vi "Operational Force Test SAA.vi"(8 "error in (no error)":errorcluster, 10 "Model in":refnum<class "Model.lvclass">, 11 "Test Actuator State in":refnum<class "Test Actuator State.lvclass">) -> (0 "error out":errorcluster, 1 "Pass":bool, 2 "Model out":refnum<class "Model.lvclass">, 3 "Test Actuator State out":refnum<class "Test Actuator State.lvclass">)   [LabVIEW 2016]
uses:
  Model/Model/Model.lvclass
  Typedefs/ActuatorSetPoints.ctl
  <vilib>/platform/TimedLoop/XDataNode/XDataNode.xnode
  <vilib>/Platform/TimedLoop/XDataNode/nitl_modes.ctl
  <vilib>/Platform/TimedLoop/XDataNode/XDNodeRunTimeDep.lvlib
  <vilib>/Platform/TimedLoop/XDataNode/wakeup.ctl
  <vilib>/Platform/TimedLoop/XDataNode/timing_clust.ctl
  Test Actuator State.lvclass
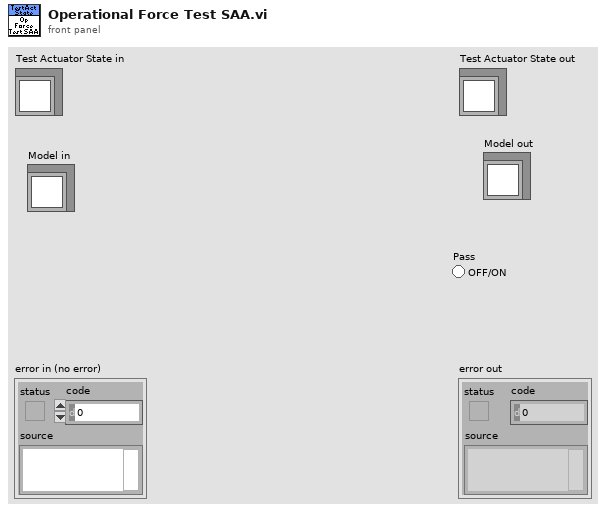
[diagram p1: front panel]
types:
  T1 = typedef "ForcePair.ctl" = cluster{"Axial Force":dbl, "Lateral Force":dbl}
  T2 = typedef "OperationalForceTestSettings.ctl" = cluster{"Max Force Error (N)":dbl, "Max Moment (NM)":dbl, "Process Time (s)":dbl, "Sample Time (s)":dbl}
  T3 = typedef "ActuatorSetPoints.ctl" = cluster{"Axial Force":dbl, "Lateral Force":dbl, "FC1 Force":dbl, "FC2 Force":dbl}
  T4 = typedef "XDNodeRunTimeDep.lvlib/timing_clust.ctl" = cluster{"Expected End [f-1]":u64, "Actual End [f-1]":u64, "Finished Late? [f-1]":bool, "Expected End [i-1]":u64, "Actual End [i-1]":u64, "Finished Late? [i-1]":bool, "Expected Start [i]":u64, "Actual Start [i]":u64, "Expected Start [f]":u64, "Actual Start [f]":u64, "Source Name":string, "Structure Name":string, "Period":i64, "Deadline":i64, "Offset":i64, "Start":i64, "Priority":i32, "Timeout":i32, "Mode":T5, "Wakeup Reason":T6, "Error":errorcluster, "Source Type":string, "Secondary Source Type":string, "Global End Time":u64, "Global Start Time":u64, "Frame Duration":u64, "Iteration Duration":u64, "Assigned CPU":i32, "I/O Scan Engine Mode":u32}
  T5 = typedef "XDNodeRunTimeDep.lvlib/nitl_modes.ctl" = enum32{"No Change", "Process missed periods, maintain original phase", "Discard missed periods, maintain original phase", "Process missed periods, ignore original phase", "Discard missed periods, ignore original phase"}
  T6 = typedef "XDNodeRunTimeDep.lvlib/wakeup.ctl" = enum32{"Normal", "Aborted", "Asynchronous wakeup", "Timing source error", "Timed loop error", "Timeout"}
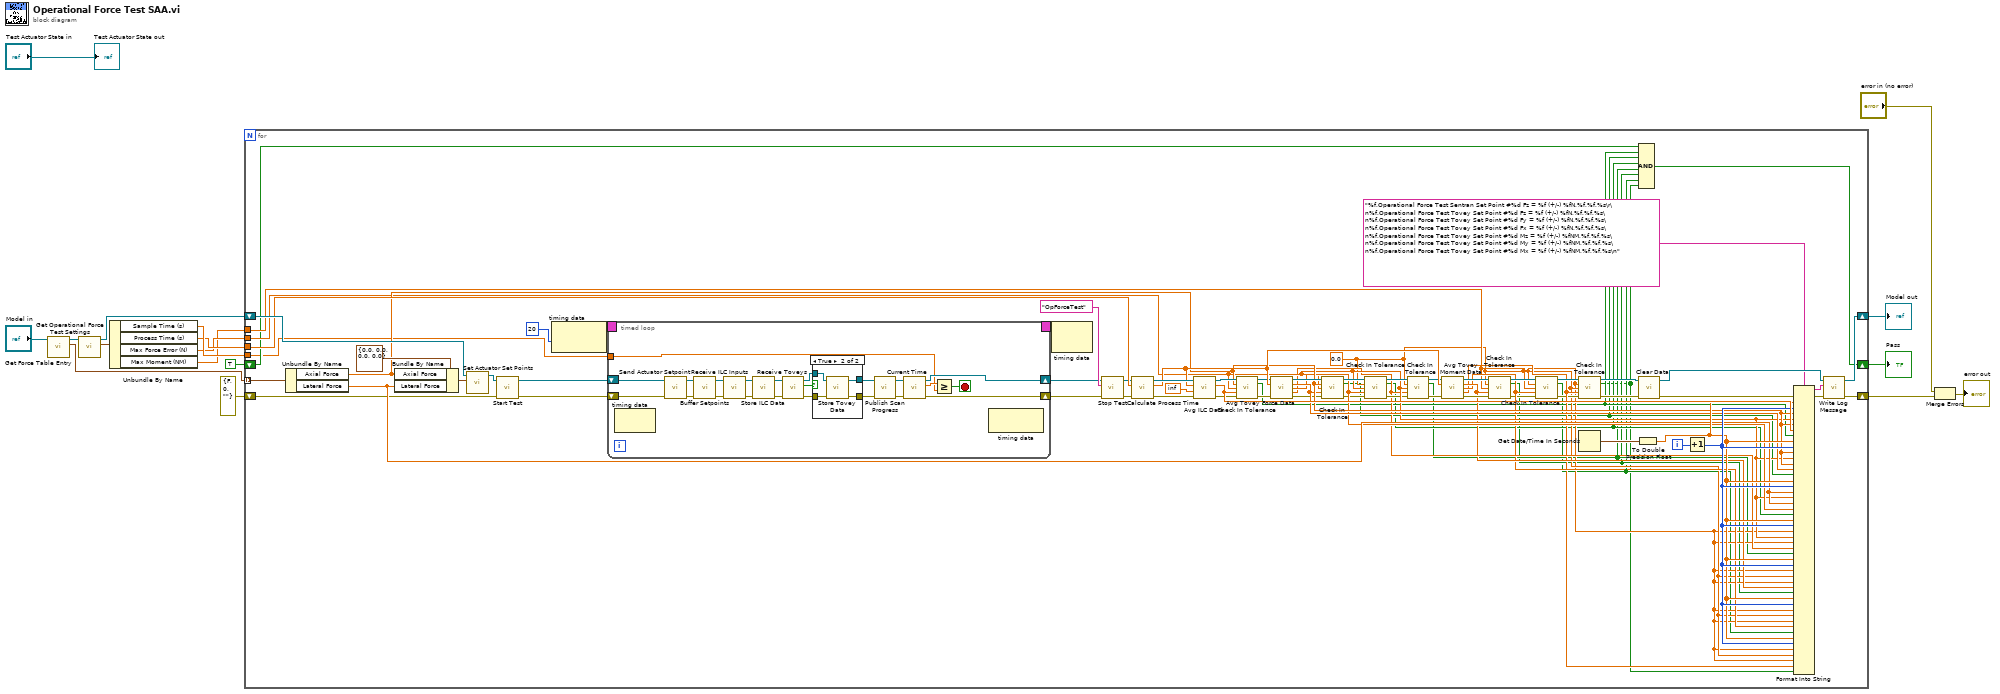
[diagram p0: block diagram]
diagram:
  n1 = call "Get Force Table Entry.vi"("Model in"="Model in") -> ("Entry"=w4:T1[], "Model out"=w7:refnum<class "Model.lvclass">)  [unwired: 8 in, 1 out]
  n2 = call-dynamic "Get Operational Force Test Settings.vi"("Model in"=w7) -> ("Operational Force Test Settings"=w5:T2, "Model out"=w6:refnum<class "Model.lvclass">)  [unwired: 9 in]
  n3 = Unbundle By Name(w5) -> ("Sample Time (s)"=w16:dbl, "Process Time (s)"=w15:dbl, "Max Force Error (N)"=w14:dbl, "Max Moment (NM)"=w9:dbl)
  n4 = for {
    tunnel: w4 -> [w83] mode=indexing
    shift-right: [w88] -> w11
    shift-left: w6 -> [w90]
    tunnel: w16 -> [w22]
    tunnel: w15 -> [w78]
    tunnel: w14 -> [w62]
    shift-right: [w79] -> w10
    shift-left: errorcluster {"status"=FALSE, "code"=0, "source"=""} ("error out") -> [w39]
    tunnel: w9 -> [w44]
    shift-right: [w29] -> w1
    shift-left: TRUE -> [w37]
    i -> [w85]
    w43 = 0.0
    n5 = Unbundle By Name(w83) -> ("Axial Force"=w68:dbl, "Lateral Force"=w65:dbl)
    n6 = Bundle By Name(cluster=T3 {"Axial Force"=0.0, "Lateral Force"=0.0, "FC1 Force"=0.0, "FC2 Force"=0.0} ("Actuator Set Points"), "Axial Force"=w68, "Lateral Force"=w65) -> (w84:T3)
    n7 = call "Set Actuator Set Points.vi"("Actuator Set Points"=w84, "Model in"=w90) -> ("Model out"=w38:refnum<class "Model.lvclass">)  [unwired: 9 in]
    n8 = call "Start Test.vi"("error in (no error)"=w39, "Model in"=w38) -> ("error out"=w20:errorcluster, "Model out"=w21:refnum<class "Model.lvclass">)  [unwired: 8 in]
    n9 = node-c288(i64 20 ("Period")) -> (w25:T4)
    n10 = timed-loop {
      timing: w25 -> [_]
      timing-out: [_] -> w24
      shift-right: [w95] -> w18
      shift-left: w20 -> [w96]
      shift-right: [w93] -> w19
      shift-left: w21 -> [w94]
      tunnel: w22 -> [w92]
      stop <- w97 stop-if-true
      n11 = node-c288() -> ()  [unwired: 1 in, 1 out]
      n12 = call "Send Actuator Setpoint.vi"("error in (no error)"=w96, "Model in"=w94) -> ("error out"=w112:errorcluster, "Model out"=w110:refnum<class "Model.lvclass">)  [unwired: 8 in]
      n13 = call "Buffer Setpoints.vi"("error in (no error)"=w112, "Model in"=w110) -> ("error out"=w113:errorcluster, "Model out"=w111:refnum<class "Model.lvclass">)  [unwired: 8 in]
      n14 = call "Receive ILC Inputs.vi"("error in (no error)"=w113, "Model in"=w111) -> ("error out"=w99:errorcluster, "Model out"=w98:refnum<class "Model.lvclass">)  [unwired: 8 in]
      n15 = call "Store ILC Data.vi"("error in (no error)"=w99, "Model in"=w98) -> ("error out"=w102:errorcluster, "Model out"=w101:refnum<class "Model.lvclass">)  [unwired: 8 in]
      n16 = call "Receive Toveys.vi"("error in (no error)"=w102, "Model in"=w101) -> ("error out"=w104:errorcluster, "Data Received"=w105:bool, "Model out"=w103:refnum<class "Model.lvclass">)  [unwired: 7 in]
      n17 = case shown="True" w105 {
        tunnel: w103 -> [w115 w119]
        tunnel: w104 -> [w114 w118]
        tunnel: [w114 w117] -> w109
        tunnel: [w115 w116] -> w106
        frame False {
        }
        frame True {
          n18 = call "Store Tovey Data.vi"("error in (no error)"=w118, "Model in"=w119) -> ("error out"=w117:errorcluster, "Model out"=w116:refnum<class "Model.lvclass">)  [unwired: 8 in]
        }
      }
      n19 = call "Publish Scan Progress.vi"("error in (no error)"=w109, "Model in"=w106) -> ("error out"=w108:errorcluster, "Model out"=w107:refnum<class "Model.lvclass">)  [unwired: 8 in]
      n20 = call "Current Time.vi"("error in (no error)"=w108, "Model in"=w107) -> ("error out"=w95:errorcluster, "Time"=w100:dbl, "Model out"=w93:refnum<class "Model.lvclass">)  [unwired: 7 in]
      n21 = Greater Or Equal?(x=w100, y=w92) -> (x >= y?=w97:bool)
      n22 = node-c288() -> ()  [unwired: 1 in, 1 out]
    }
    n23 = node-c288(w24) -> ()  [unwired: 1 out]
    n24 = call "Stop Test.vi"("error in (no error)"=w18, "Test"="OpForceTest", "Model in"=w19) -> ("error out"=w27:errorcluster, "Model out"=w28:refnum<class "Model.lvclass">)  [unwired: 7 in]
    n25 = call "Calculate Process Time.vi"("error in (no error)"=w27, "Seconds"=w78, "Model in"=w28) -> ("error out"=w76:errorcluster, "Time"=w75:dbl, "Model out"=w77:refnum<class "Model.lvclass">)  [unwired: 6 in]
    n26 = call "Avg ILC Data.vi"("error in (no error)"=w76, "Before This Time"=inf, "After This Time"=w75, "Model in"=w77) -> ("error out"=w72:errorcluster, "Force"=w73:dbl, "Model out"=w74:refnum<class "Model.lvclass">)  [unwired: 5 in]
    n27 = call "Check In Tolerance.vi"("Model in"=w74, "Expected"=w68, "Tolerance"=w62, "Actual"=w73, "error in (no error)"=w72) -> ("Model out"=w42:refnum<class "Model.lvclass">, "Pass"=w36:bool, "error out"=w41:errorcluster)  [unwired: 8 in]
    n28 = call "Avg Tovey Force Data.vi"("Model in"=w42, "After This Time"=w75, "error in (no error)"=w41) -> ("Model out"=w69:refnum<class "Model.lvclass">, "Fz"=w67:dbl, "Fy"=w64:dbl, "Fx"=w54:dbl, "error out"=w61:errorcluster)  [unwired: 8 in]
    n29 = call "Check In Tolerance.vi"("Model in"=w69, "Expected"=w68, "Tolerance"=w62, "Actual"=w67, "error in (no error)"=w61) -> ("Model out"=w66:refnum<class "Model.lvclass">, "Pass"=w35:bool, "error out"=w60:errorcluster)  [unwired: 8 in]
    n30 = call "Check In Tolerance.vi"("Model in"=w66, "Expected"=w43, "Tolerance"=w62, "Actual"=w64, "error in (no error)"=w60) -> ("Model out"=w63:refnum<class "Model.lvclass">, "Pass"=w34:bool, "error out"=w59:errorcluster)  [unwired: 8 in]
    n31 = call "Check In Tolerance.vi"("Model in"=w63, "Expected"=w43, "Tolerance"=w62, "Actual"=w54, "error in (no error)"=w59) -> ("Model out"=w57:refnum<class "Model.lvclass">, "Pass"=w33:bool, "error out"=w58:errorcluster)  [unwired: 8 in]
    n32 = call "Avg Tovey Moment Data.vi"("Model in"=w57, "After This Time"=w75, "error in (no error)"=w58) -> ("Model out"=w56:refnum<class "Model.lvclass">, "Mz"=w53:dbl, "My"=w50:dbl, "Mx"=w49:dbl, "error out"=w55:errorcluster)  [unwired: 8 in]
    n33 = call "Check In Tolerance.vi"("Model in"=w56, "Expected"=w43, "Tolerance"=w44, "Actual"=w53, "error in (no error)"=w55) -> ("Model out"=w52:refnum<class "Model.lvclass">, "Pass"=w32:bool, "error out"=w47:errorcluster)  [unwired: 8 in]
    n34 = call "Check In Tolerance.vi"("Model in"=w52, "Expected"=w43, "Tolerance"=w44, "Actual"=w50, "error in (no error)"=w47) -> ("Model out"=w51:refnum<class "Model.lvclass">, "Pass"=w31:bool, "error out"=w46:errorcluster)  [unwired: 8 in]
    n35 = call "Check In Tolerance.vi"("Model in"=w51, "Expected"=w43, "Tolerance"=w44, "Actual"=w49, "error in (no error)"=w46) -> ("Model out"=w48:refnum<class "Model.lvclass">, "Pass"=w30:bool, "error out"=w45:errorcluster)  [unwired: 8 in]
    n36 = Get Date/Time In Seconds() -> (seconds since 1Jan1904=w86:timestamp)
    n37 = To Double Precision Float(number=w86) -> (double precision float=w70:dbl)
    n38 = call "Clear Data.vi"("error in (no error)"=w45, "Model in"=w48) -> ("error out"=w81:errorcluster, "Model out"=w89:refnum<class "Model.lvclass">)  [unwired: 8 in]
    n39 = Compound Arithmetic op=AND(w37, w36, w35, w34, w33, w32, w31, w30) -> (w29:bool)
    n40 = Increment(x=w85) -> (x+1=w71:i32)
    n41 = Format Into String(format string="%f,Operational Force Test Sentran Set Point #%d Fz = %f (+/-) %fN,%f,%f,%s\r\n%f,Operational Force Test Tovey Set Point #%d Fz = %f (+/-) %fN,%f,%f,%s\n%f,Operational Force Test Tovey Set Point #%d Fy = %f (+/-) %fN,%f,%f,%s\n%f,Operational Force Test Tovey Set Point #%d Fx = %f (+/-) %fN,%f,%f,%s\n%f,Operational Force Test Tovey Set Point #%d Mz = %f (+/-) %fNM,%f,%f,%s\n%f,Operational Force Test Tovey Set Point #%d My = %f (+/-) %fNM,%f,%f,%s\n%f,Operational Force Test Tovey Set Point #%d Mx = %f (+/-) %fNM,%f,%f,%s\n", error in=w81, w70, w71, w68, w62, w68, w73, w36, w70, w71, w68, w62, w68, w67, w35, w70, w71, w65, w62, w65, w64, w34, w70, w71, w43, w62, w43, w54, w33, w70, w71, w43, w44, w43, w53, w32, w70, w71, w43, w44, w43, w50, w31, w70, w71, w43, w44, w43, w49, w30) -> (resulting string=w82:string, error out=w80:errorcluster)  [unwired: 1 in]
    n42 = call "Write Log Message.vi"("error in (no error)"=w80, "Message"=w82, "Model in"=w89) -> ("error out"=w79:errorcluster, "Model out"=w88:refnum<class "Model.lvclass">)  [unwired: 7 in]
  }
  "Model out" <- w11
  "Pass" <- w1
  n43 = Merge Errors("error in (no error)", w10) -> (→"error out":errorcluster)
  "Test Actuator State out" <- "Test Actuator State in"
